vi "Shared Variables CD 2.0 RT Driver VI.vi"(7 "Operation":T1, 11 "Device Reference in":T2 format="%.0x") -> (0 "Error Code":i32)   [LabVIEW 2020, in "Shared Variables CD 2.0 Engine.lvlib"]
uses:
  Shared Variables CD 2.0 Engine.lvlib
  <vilib>/NI VeriStand/Custom Device API/Custom Device Item Ref.ctl
  <vilib>/NI VeriStand/Custom Device API/Hardware Interface Driver VI Operation.ctl
  <vilib>/NI VeriStand/Custom Device API/Block Data Reference.ctl
  <vilib>/NI VeriStand/Custom Device API/Data Reference.ctl
  Shared DataTypes/SV Process Data.ctl
  Shared DataTypes/URLs.ctl
  <vilib>/NI VeriStand/Custom Device API/Data Access Type.ctl
  Shared/Shared Variables CD 2.0 GUID Lookup.vi
  <vilib>/NI VeriStand/Custom Device API/Global Data Refs.vi
  <vilib>/NI VeriStand/Custom Device API/Custom Device API.lvlib
  <vilib>/NI VeriStand/Custom Device Tools/Custom Device Utility Library/Custom Device Utility Library.lvlib
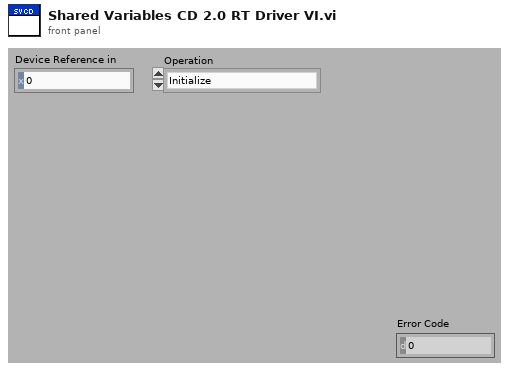
[diagram p1: front panel]
types:
  T1 = typedef "Custom Device API.lvlib/Hardware Interface Driver VI Operation.ctl" = enum16{"Initialize", "Start", "Read Data from HW", "Write Data to HW", "Close"}
  T2 = typedef "Custom Device API.lvlib/Custom Device Item Ref.ctl" = u64
  T3 = typedef "Custom Device API.lvlib/Block Data Reference.ctl" = cluster{"Data Reference":T4, "Offset":u64, "Length":u64}
  T4 = typedef "Custom Device API.lvlib/Data Reference.ctl" = i32
  T5 = typedef "SV Process Data.ctl" = cluster{"Write URLs":T6, "Read URLs":T6, "Write SV FIFO":string, "Read SV FIFO":string, "Status SV FIFO":string, "Status Notifier":string, "Update Rate":u32}
  T6 = typedef "URLs.ctl" = cluster{"URLs":string[]}
  T7 = cluster{"Output Ref":cluster{"Block Data Refs":T3[], "Values Array":dbl[]}, "Input Ref":cluster{"Block Data Refs":T3[], "Values Array":dbl[]}, "Status Ref":cluster{"Block Data Refs":T3[], "Values Array":dbl[]}, "Write FIFO":refnum<k33>, "Read FIFO":refnum<k33>, "Status FIFO":refnum<k33>, "Status":refnum<notifier>, "Process Data":T5, "Device Error":errorcluster}
  T8 = typedef "Custom Device API.lvlib/Data Access Type.ctl" = enum16{"Read", "Write"}
  T9 = cluster{"Block Data Refs":T3[], "Values Array":dbl[]}
  T10 = typedef "Custom Device API.lvlib/Custom Device Target Type.ctl" = enum16{"PharLap", "VxWorks", "Windows", "Linux_32_ARM", "Linux_x64"}
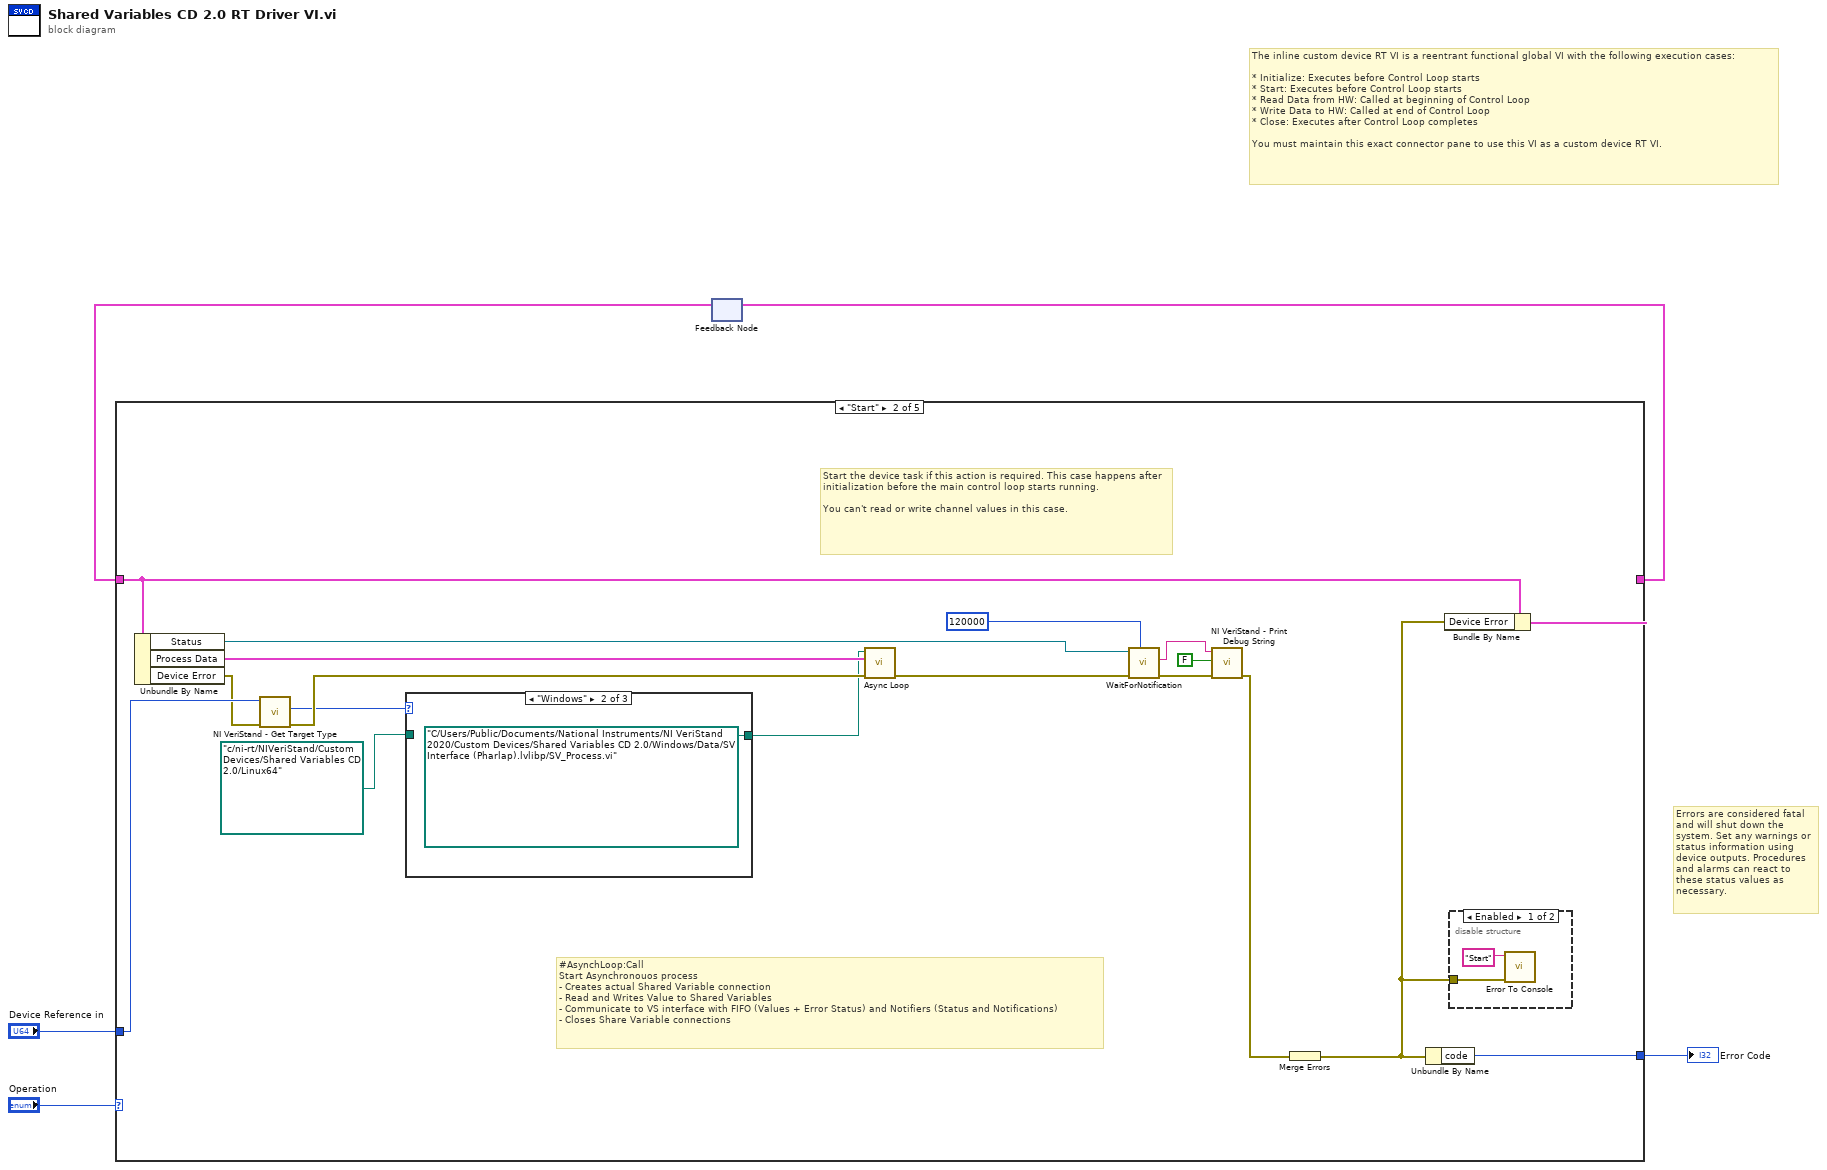
[diagram p0: block diagram]
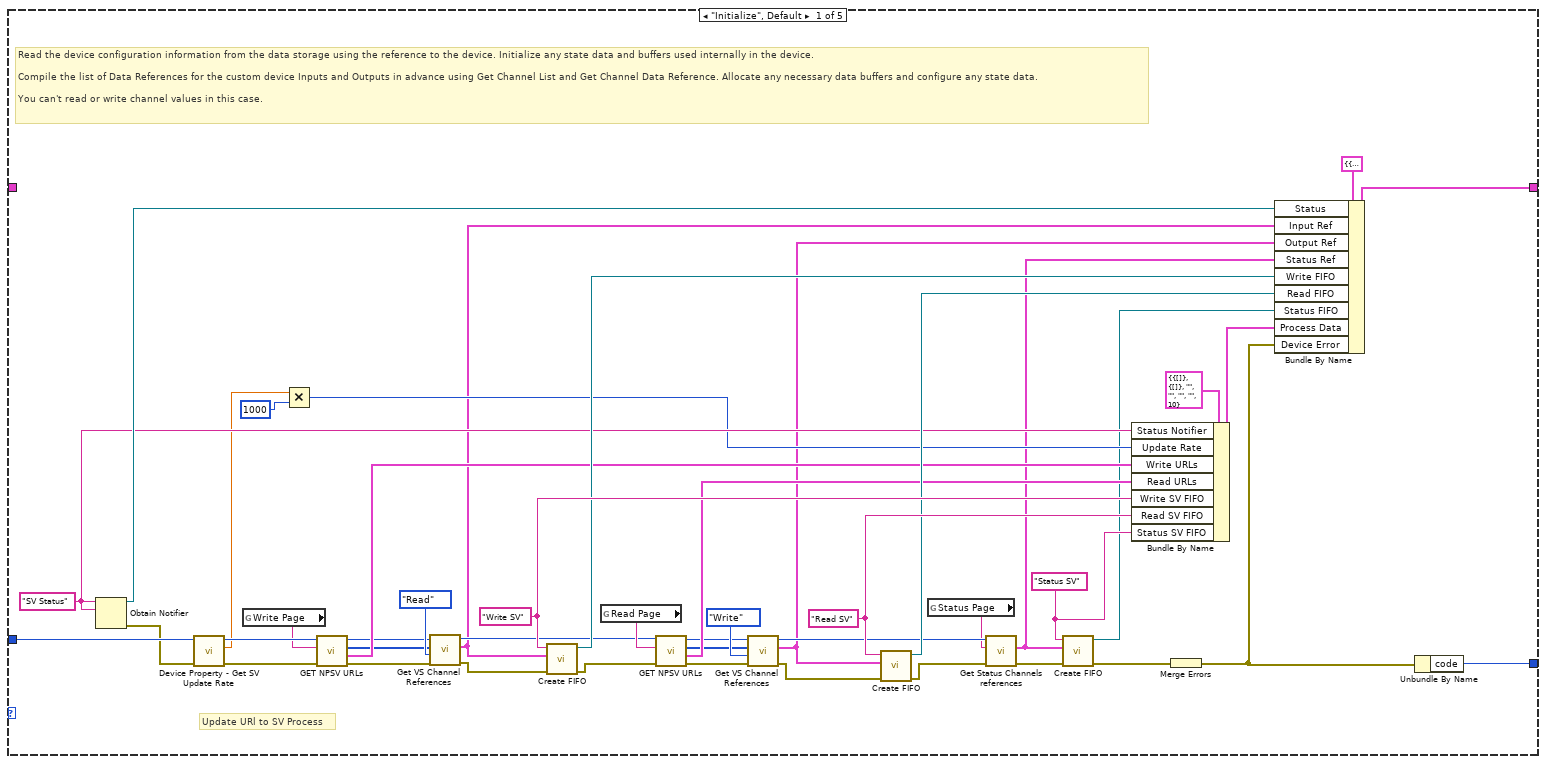
[diagram p2: hidden frame]
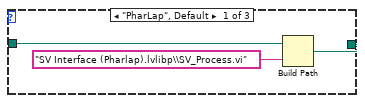
[diagram p3: hidden frame]
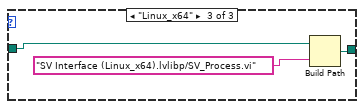
[diagram p4: hidden frame]
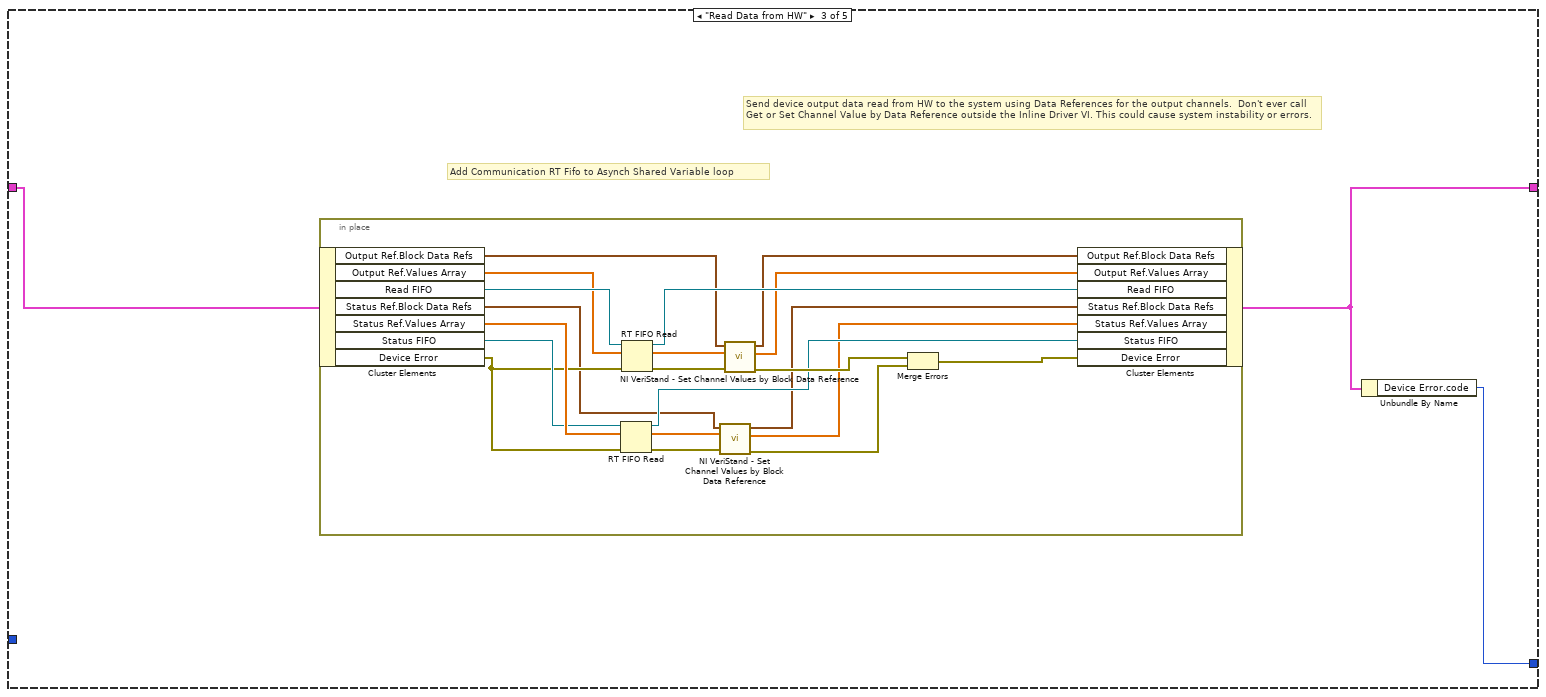
[diagram p6: hidden frame]
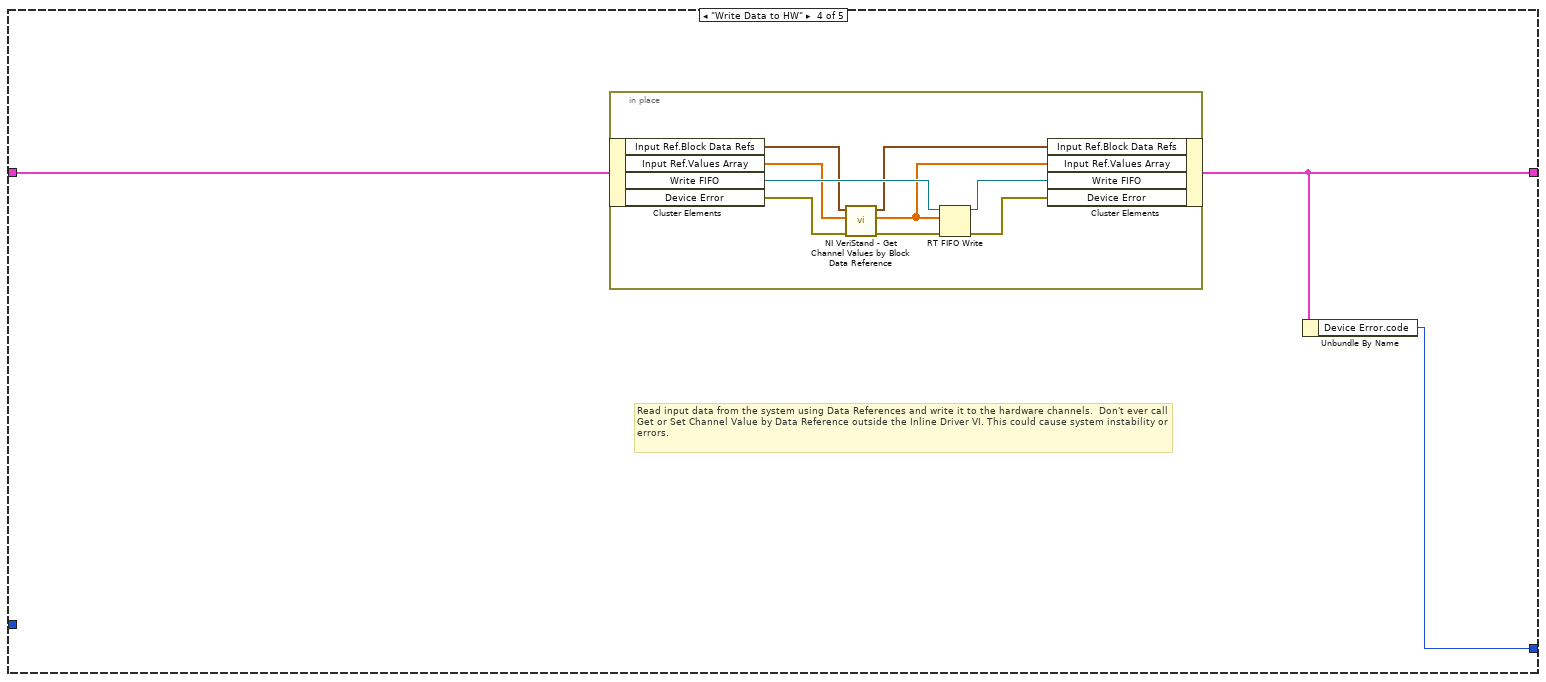
[diagram p7: hidden frame]
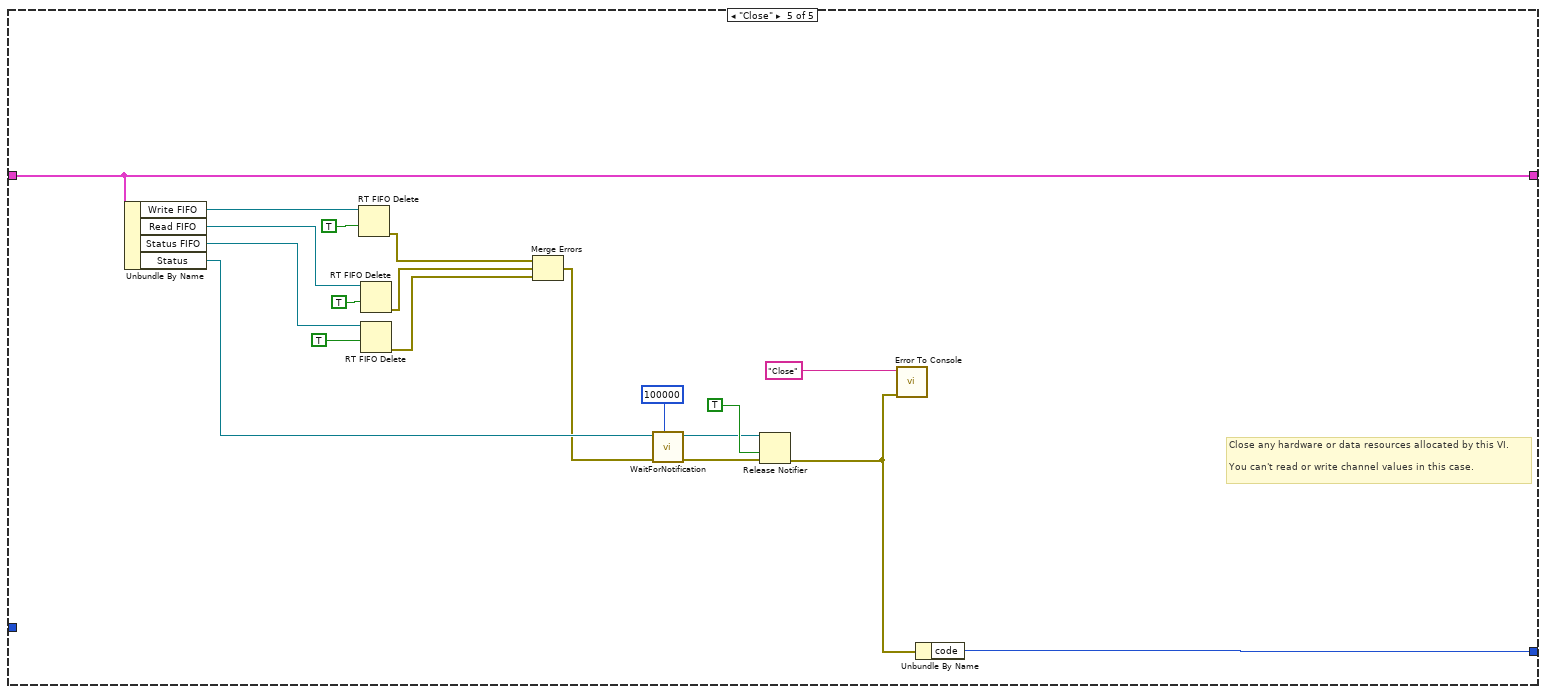
[diagram p8: hidden frame]
diagram:
  # "Errors are considered fatal and will shut down the system. Set any warnings or status information using device outputs. Procedures and alarms can react to these status values as necessary."
  # "The inline custom device RT VI is a reentrant functional global VI with the following execution cases:\n\n* Initialize: Executes before Control Loop starts\n* Start: Executes before Control Loop starts\n* Read Data from HW: Called at beginning of Control Loop\n* Write Data to HW: Called at end of Control Loop\n* Close: Executes after Control Loop completes\n\nYou must maintain this exact connector pane to use this VI as a custom device RT VI."
  n1 = feedback #1() -> (w3:T7)  [unwired: 1 out]
  n2 = case shown="\"Start\"" "Operation" {
    tunnel: [w50 w67 w79 w102 w130] -> w4
    tunnel: w3 -> [_ w58 w80 w103 w130]
    tunnel: "Device Reference in" -> [w43 w56 _ _ _]
    tunnel: [w48 w68 w78 w101 w131] -> w1
    frame "Initialize", Default {
      w19 = "Status SV" ("FIFO Name")
      w27 = "SV Status" ("name (unnamed)")
      w36 = "Write SV" ("FIFO Name")
      w37 = "Read SV" ("name (unnamed)")
      # "Update URl to SV Process"
      # "Read the device configuration information from the data storage using the reference to the device. Initialize any state data and buffers used internally in the device.\n\nCompile the list of Data References for the custom device Inputs and Outputs in advance using Get Channel List and Get Channel Data Reference. Allocate any necessary data buffers and configure any state data.\n\nYou can't read or write channel values in this case."
      n3 = Obtain Notifier(name (unnamed)=w27, notification data type=w27) -> (notifier out=w45:refnum<notifier>, error out=w41:errorcluster)  [unwired: 2 in, 1 out]
      n4 = call "Device Property - Get SV Update Rate.vi"("error in (no error)"=w41, "Device Ref in"=w43) -> ("error out"=w40:errorcluster, "Update Rate (ms)"=w26:dbl, "Device Ref out"=w42:T2)  [unwired: 7 in]
      n5 = global read "Shared Variables CD 2.0 GUID Lookup.vi" "Write Page"() -> (w32:string)
      n6 = Multiply(x=w26, y=u32 1000) -> (x*y=w25:u32)
      n7 = call "GET NPSV URLs.vi"("error in (no error)"=w40, "Page"=w32, "Device Reference in"=w42) -> ("error out"=w13:errorcluster, "SV"=w31:T6, "Channel Refs"=w30:T2[], "Device Reference out"=w14:T2)  [unwired: 5 in]
      n8 = call "Get VS Channel References.vi"("error in (no error)"=w13, "Access (Read)"=Data_Access_Type."Read" ("Access"), "Channel Refs"=w30, "Device Reference in"=w14) -> ("error out"=w12:errorcluster, "DataRef"=w7:T9, "Device Reference out"=w15:T2)  [unwired: 5 in]
      n9 = call "Create FIFO.vi"("error in (no error)"=w12, "DataRef"=w7, "FIFO Name"=w36) -> ("error out"=w11:errorcluster, "FIFO Ref"=w34:refnum<k33>)  [unwired: 7 in]
      n10 = global read "Shared Variables CD 2.0 GUID Lookup.vi" "Read Page"() -> (w33:string)
      n11 = call "GET NPSV URLs.vi"("error in (no error)"=w11, "Page"=w33, "Device Reference in"=w15) -> ("error out"=w17:errorcluster, "SV"=w29:T6, "Channel Refs"=w28:T2[], "Device Reference out"=w16:T2)  [unwired: 5 in]
      n12 = call "Get VS Channel References.vi"("error in (no error)"=w17, "Access (Read)"=Data_Access_Type."Write" ("Access"), "Channel Refs"=w28, "Device Reference in"=w16) -> ("error out"=w10:errorcluster, "DataRef"=w6:T9, "Device Reference out"=w22:T2)  [unwired: 5 in]
      n13 = call "Create FIFO.vi"("error in (no error)"=w10, "DataRef"=w6, "FIFO Name"=w37) -> ("error out"=w9:errorcluster, "FIFO Ref"=w35:refnum<k33>)  [unwired: 7 in]
      n14 = global read "Shared Variables CD 2.0 GUID Lookup.vi" "Status Page"() -> (w21:string)
      n15 = call "Get Status Channels references.vi"("error in (no error)"=w9, "Page"=w21, "Device Reference in"=w22) -> ("error out"=w8:errorcluster, "Status Ref"=w20:T9)  [unwired: 6 in, 1 out]
      n16 = call "Create FIFO.vi"("error in (no error)"=w8, "DataRef"=w20, "FIFO Name"=w19) -> ("error out"=w23:errorcluster, "FIFO Ref"=w18:refnum<k33>)  [unwired: 7 in]
      n17 = Bundle By Name(cluster=T5 {"Write URLs"={"URLs"=[]}, "Read URLs"={"URLs"=[]}, "Write SV FIFO"="", "Read SV FIFO"="", "Status SV FIFO"="", "Status Notifier"="", "Update Rate"=10} ("Cluster"), "Status Notifier"=w27, "Update Rate"=w25, "Write URLs"=w31, "Read URLs"=w29, "Write SV FIFO"=w36, "Read SV FIFO"=w37, "Status SV FIFO"=w19) -> (w38:T5)
      n18 = Merge Errors(w23) -> (w44:errorcluster)
      n19 = Bundle By Name(cluster=T7 {"Output Ref"={"Block Data Refs"=[], "Values Array"=[]}, "Input Ref"={"Block Data Refs"=[], "Values Array"=[]}, "Status Ref"={"Block Data Refs"=[], "Values Array"=[]}, "Write FIFO"=refnum, "Read FIFO"=refnum, "Status FIFO"=refnum, "Status"=refnum, "Process Data"={"Write URLs"={"URLs"=[]}, "Read URLs"={"URLs"=[]}, "Write SV FIFO"="", "Read SV FIFO"="", "Status SV FIFO"="", "Status Notifier"="", "Update Rate"=10}, "Device Error"={"status"=FALSE, "code"=0, "source"=""}}, "Status"=w45, "Input Ref"=w7, "Output Ref"=w6, "Status Ref"=w20, "Write FIFO"=w34, "Read FIFO"=w35, "Status FIFO"=w18, "Process Data"=w38, "Device Error"=w44) -> (w50:T7)
      n20 = Unbundle By Name(w44) -> ("code"=w48:i32)
    }
    frame "Start" {
      # "#AsynchLoop:Call\nStart Asynchronouos process\n- Creates actual Shared Variable connection\n- Read and Writes Value to Shared Variables\n- Communicate to VS interface with FIFO (Values + Error Status) and Notifiers (Status and Notifications)\n- Closes Share Variable connections"
      # "Start the device task if this action is required. This case happens after initialization before the main control loop starts running.\n\nYou can't read or write channel values in this case."
      n21 = Unbundle By Name(w58) -> ("Status"=w66:refnum<notifier>, "Process Data"=w59:T5, "Device Error"=w55:errorcluster)
      n22 = call <vilib>:"NI VeriStand - Get Target Type.vi"("error in (no error)"=w55, "Item Ref in"=w56) -> ("error out"=w54:errorcluster, "Target Type"=w52:T10)  [unwired: 7 in, 1 out]
      n23 = case shown="\"Windows\"" w52 {
        tunnel: path "c:/ni-rt/NIVeriStand/Custom Devices/Shared Variables CD 2.0/Linux64" -> [w70 _ w74]
        tunnel: [w69 path "C:/Users/Public/Documents/National Instruments/NI VeriStand 2020/Custom Devices/Shared Variables CD 2.0/Windows/Data/SV Interface (Pharlap).lvlibp/SV_Process.vi" w73] -> w51
        frame "PharLap", Default {
          n24 = Build Path(base path=w70, name or relative path="SV Interface (Pharlap).lvlibp\\SV_Process.vi") -> (appended path=w69:path)
        }
        frame "Windows" {
        }
        frame "Linux_x64" {
          n25 = Build Path(base path=w74, name or relative path="SV Interface (Linux_x64).lvlibp/SV_Process.vi") -> (appended path=w73:path)
        }
      }
      n26 = call "Async Loop.vi"("error in (no error)"=w54, "Process Data"=w59, "Path"=w51) -> ("error out"=w60:errorcluster)  [unwired: 8 in]
      n27 = call "WaitForNotification.vi"("timeout in ms (-1)"=120000, "error in (no error)"=w60, "Notifier in"=w66) -> ("error out"=w63:errorcluster, "Status out"=w62:string)  [unwired: 6 in, 1 out]
      n28 = call <vilib>:"NI VeriStand - Print Debug String.vi"("error in (no error)"=w63, "Add to log file? (F)"=FALSE ("Add to log file? (T)"), "Message"=w62) -> ("error out"=w57:errorcluster)  [unwired: 8 in]
      n29 = Merge Errors(w57) -> (w64:errorcluster)
      n30 = Unbundle By Name(w64) -> ("code"=w68:i32)
      n31 = Bundle By Name(cluster=w58, "Device Error"=w64) -> (w67:T7)
      n32 = disable-structure shown="Enabled" {
        disable-tunnel: w64 -> [w77 _]
        frame Enabled {
          n33 = call "Error To Console.vi"("error in (no error)"=w77, "Add Text to Message"="Start") -> ()  [unwired: 10 in]
        }
        frame Disabled {
        }
      }
    }
    frame "Read Data from HW" {
      # "Add Communication RT Fifo to Asynch Shared Variable loop"
      # "Send device output data read from HW to the system using Data References for the output channels.  Don't ever call Get or Set Channel Value by Data Reference outside the Inline Driver VI. This could cause system instability or errors."
      n34 = in-place {
        n35 = in-place-cluster #2(w80) -> ("Output Ref.Block Data Refs"=w94:T3[], "Output Ref.Values Array"=w96:dbl[], "Read FIFO"=w100:refnum<k33>, "Status Ref.Block Data Refs"=w84:T3[], "Status Ref.Values Array"=w91:dbl[], "Status FIFO"=w90:refnum<k33>, "Device Error"=w89:errorcluster)
        n36 = RT FIFO Read(0:w90, 1:w91, 3:w89) -> (8:w87:refnum<k33>, 9:w86:dbl[], 11:w88:errorcluster)  [unwired: 1 in, 2 out]
        n37 = RT FIFO Read(0:w100, 1:w96, 3:w89) -> (8:w97:refnum<k33>, 9:w99:dbl[], 11:w98:errorcluster)  [unwired: 1 in, 2 out]
        n38 = call <vilib>:"NI VeriStand - Set Channel Values by Block Data Reference.vi"("error in (no error)"=w88, "Values Array in"=w86, "Block Data Ref"=w84) -> ("error out"=w81:errorcluster, "Values Array out"=w85:dbl[], "Block Data Ref dup"=w83:T3[])  [unwired: 6 in]
        n39 = call <vilib>:"NI VeriStand - Set Channel Values by Block Data Reference.vi"("error in (no error)"=w98, "Values Array in"=w99, "Block Data Ref"=w94) -> ("error out"=w92:errorcluster, "Values Array out"=w95:dbl[], "Block Data Ref dup"=w93:T3[])  [unwired: 6 in]
        n40 = Merge Errors(w92, w81) -> (w82:errorcluster)
        n41 = in-place-cluster #2("Output Ref.Block Data Refs"=w93, "Output Ref.Values Array"=w95, "Read FIFO"=w97, "Status Ref.Block Data Refs"=w83, "Status Ref.Values Array"=w85, "Status FIFO"=w87, "Device Error"=w82) -> (w79:T7)
      }
      n42 = Unbundle By Name(w79) -> ("Device Error.code"=w78:i32)
    }
    frame "Write Data to HW" {
      # "Read input data from the system using Data References and write it to the hardware channels.  Don't ever call Get or Set Channel Value by Data Reference outside the Inline Driver VI. This could cause system instability or errors."
      n43 = in-place {
        n44 = in-place-cluster #3(w103) -> ("Input Ref.Block Data Refs"=w107:T3[], "Input Ref.Values Array"=w108:dbl[], "Write FIFO"=w109:refnum<k33>, "Device Error"=w112:errorcluster)
        n45 = call <vilib>:"NI VeriStand - Get Channel Values by Block Data Reference.vi"("error in (no error)"=w112, "Values Array in"=w108, "Block Data Ref"=w107) -> ("error out"=w111:errorcluster, "Values Array out"=w105:dbl[], "Block Data Ref dup"=w106:T3[])  [unwired: 6 in]
        n46 = RT FIFO Write(0:w109, 1:w105, 3:w111) -> (8:w104:refnum<k33>, 11:w110:errorcluster)  [unwired: 2 in, 2 out]
        n47 = in-place-cluster #3("Input Ref.Block Data Refs"=w106, "Input Ref.Values Array"=w105, "Write FIFO"=w104, "Device Error"=w110) -> (w102:T7)
      }
      n48 = Unbundle By Name(w102) -> ("Device Error.code"=w101:i32)
    }
    frame "Close" {
      # "Close any hardware or data resources allocated by this VI.\n\nYou can't read or write channel values in this case."
      n49 = Unbundle By Name(w130) -> ("Write FIFO"=w116:refnum<k33>, "Read FIFO"=w118:refnum<k33>, "Status FIFO"=w115:refnum<k33>, "Status"=w126:refnum<notifier>)
      n50 = RT FIFO Delete(0:w116, 2:TRUE ("force destroy? (F)")) -> (11:w122:errorcluster)  [unwired: 1 in]
      n51 = RT FIFO Delete(0:w118, 2:TRUE ("force destroy? (F)")) -> (11:w121:errorcluster)  [unwired: 1 in]
      n52 = RT FIFO Delete(0:w115, 2:TRUE ("force destroy? (F)")) -> (11:w113:errorcluster)  [unwired: 1 in]
      n53 = Merge Errors(w122, w121, w113) -> (w120:errorcluster)
      n54 = call "WaitForNotification.vi"("timeout in ms (-1)"=100000, "error in (no error)"=w120, "Notifier in"=w126) -> ("error out"=w124:errorcluster, "Notifier out"=w125:refnum<notifier>)  [unwired: 6 in, 1 out]
      n55 = Release Notifier(notifier=w125, force destroy? (F)=TRUE, error in (no error)=w124) -> (error out=w128:errorcluster)  [unwired: 2 out]
      n56 = call "Error To Console.vi"("error in (no error)"=w128, "Add Text to Message"="Close") -> ()  [unwired: 10 in]
      n57 = Unbundle By Name(w128) -> ("code"=w131:i32)
    }
  }
  "Error Code" <- w1
  n58 = feedback-in #1(w4) -> ()
